vi "Git_ProgressWindowInit.vi"(8 "error in (no error)":errorcluster, 11 "Message":string) -> (0 "error out":errorcluster, 2 "Cancel Ref Out":refnum<vi>, 3 "Slide out":refnum<vi>)   [LabVIEW 2012]
uses:
  Git_ProgressFGV_enum.ctl
  Justin/FlexMeasure/LittleHelpers/GetControlRef/GetAllControlRefs_Ref.vi
  Justin/FlexMeasure/LittleHelpers/GetControlRef/GetControl_Slide.vi
  Justin/FlexMeasure/LittleHelpers/GetControlRef/GetControl_Boolean.vi
  Justin/FlexMeasure/LittleHelpers/GetControlRef/GetControl_String.vi
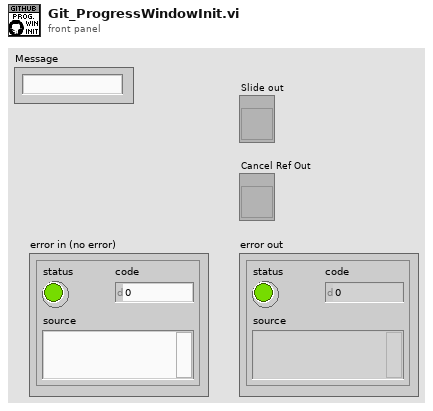
[diagram p1: front panel]
types:
  T1 = typedef "Git_ProgressFGV_enum.ctl" = enum16{"Init", "Update"}
  T2 = typedef "ControlReferences.ctl" = cluster{"Control[i]":refnum<vi>[], "Control Label Chain[i]":string[], "Control Type[i]":T3[]}
  T3 = typedef "ClassID Names Enum__ogtk.ctl" = enum32{"0 <undefined>", "1 <undefined>", "2 <undefined>", "Generic", "Decoration", "Text", "Control", "ColorBox", "Boolean", "RefNum", "Variant", "Path", "ListBox", "Table", "Array", "Picture", "ActiveXContainer", "Numeric", "Digital", "NamedNumeric", "ColorRamp", "Slide", "GraphOrChart", "WaveformChart", "WaveformGraph", "IntensityChart", "IntensityGraph", "String", "IOName", "ComboBox", "Cluster", "Panel", "Knob", "NumWithScale", "Ring", "Enum", "GObject", "Plot", "Cursor", "NumericText", "Scale", "ColorScale", "GraphScale", "ColorGraphScale", "TypedRefNum", "OldKnobScale", "MCListbox", "MeasureData", "BVTag", "DAQName", "VISAName", "IVIName", "SlideScale", "TabControl", "Page", "TabArrayTabControl", "ConPane"}
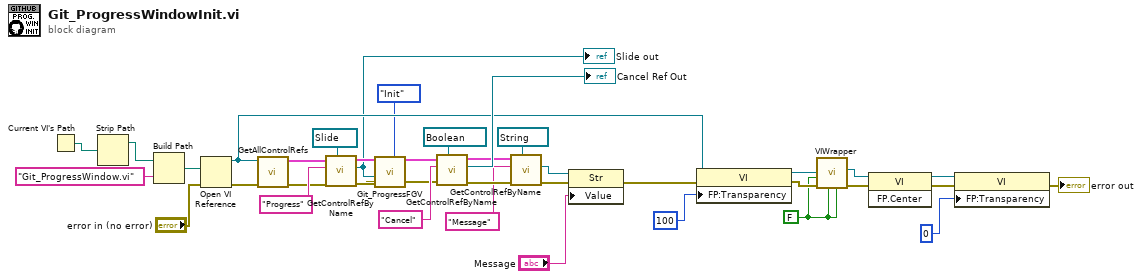
[diagram p0: block diagram]
diagram:
  w9 = FALSE ("CloseVIRef")
  n1 = Current VI's Path() -> (path=w14:path)
  n2 = Strip Path(path=w14) -> (stripped path=w15:path)  [unwired: 1 out]
  n3 = Build Path(base path=w15, name or relative path="Git_ProgressWindow.vi") -> (appended path=w17:path)
  n4 = Open VI Reference(vi path=w17, error in (no error)="error in (no error)") -> (vi reference=w31:refnum<vi>, error out=w26:errorcluster)  [unwired: 4 in]
  n5 = call-poly "GetAllControlRefs.vi"("error in (no error)"=w26, "VI Ref"=w31) -> ("error out"=w28:errorcluster, "RefCluster Out"=w27:T2)  [unwired: 8 in]
  n6 = call-poly "GetControlRefByName.vi"("Control Class"=refnum<vi> refnum, "error in (no error)"=w28, "Control Label"="Progress", "Ref Cluster In"=w27) -> ("error out"=w13:errorcluster, "Reference Out"=w10:refnum<vi>, "Ref Cluster Out"=w33:T2)  [unwired: 5 in]
  "Slide out" <- w10
  n7 = call "Git_ProgressFGV.vi"("Action"=Git_ProgressFGV_enum."Init", "Error In"=w13, "Slide in"=w10) -> ("Error Out"=w11:errorcluster)  [unwired: 8 in]
  n8 = call-poly "GetControlRefByName.vi"("Control Class"=refnum<vi> refnum, "error in (no error)"=w11, "Control Label"="Cancel", "Ref Cluster In"=w33) -> ("error out"=w7:errorcluster, "Reference Out"=→"Cancel Ref Out":refnum<vi>, "Ref Cluster Out"=w6:T2)  [unwired: 5 in]
  n9 = call-poly "GetControlRefByName.vi"("Control Class"=refnum<vi> refnum, "error in (no error)"=w7, "Control Label"="Message", "Ref Cluster In"=w6) -> ("error out"=w5:errorcluster, "Reference Out"=w2:refnum<vi>)  [unwired: 5 in, 1 out]
  n10 = property class="Str"(reference=w2, error in=w5, "Value"="Message") -> (error out=w3:errorcluster)  [unwired: 1 out]
  n11 = property class="VI"(reference=w31, error in=w3, "FP:Transparency"=u8 100 ("Front Panel Window:Transparency")) -> (reference out=w21:refnum<vi>, error out=w22:errorcluster)
  n12 = call "VIWrapper.vi"("CloseVIRef"=w9, "Wait Until Done?"=w9, "error in (no error)"=w22, "SubPanelInsert"=w9, "vi reference"=w21) -> ("error out"=w19:errorcluster, "Vi Ref out"=w18:refnum<vi>)  [unwired: 5 in]
  n13 = invoke class="VI" method="FP.Center"(reference=w18, error in=w19) -> (reference out=w23:refnum<vi>, error out=w24:errorcluster)  [unwired: 1 in, 1 out]
  n14 = property class="VI"(reference=w23, error in=w24, "FP:Transparency"=u8 0 ("Front Panel Window:Transparency")) -> (error out=→"error out":errorcluster)  [unwired: 1 out]
